vi "Scale Change for Input.vi"(0 "SP:":dbl=34.21052631578948, 1 "Slide Refnum":refnum<vi>, 2 "Slide Refnum 2":refnum<vi>, 3 "WFChart Refnum":refnum<vi>, 5 "Input Unit":enum16{"%", "EGU"}(ring), 7 "Change Scales":bool, 9 "Max In":dbl, 11 "Min In":dbl) -> (4 "SP After Scale Change":dbl=34.21052631578948)   [LabVIEW 2023]
uses:
  <vilib>/addons/control/pid/pid.llb/PID EGU to Percentage (DBL).vi
  <vilib>/addons/control/pid/pid.llb/PID Percentage to EGU (DBL).vi
  <vilib>/addons/control/pid/NI_PID_pid.lvlib
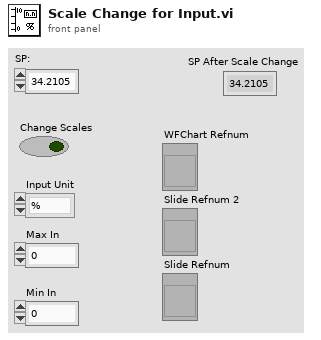
[diagram p1: front panel]
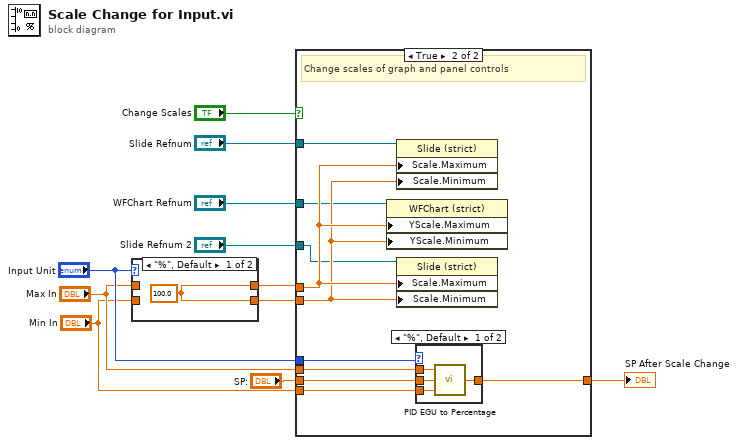
[diagram p0: block diagram]
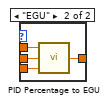
[diagram p3: hidden frame]
diagram:
  n1 = case shown="\"%\", Default" "Input Unit" {
    tunnel: [w12 w14] -> w10
    tunnel: [w12 w13] -> w11
    tunnel: "Max In" -> [_ w14]
    tunnel: "Min In" -> [_ w13]
    frame "%", Default {
      w12 = 100.0 ("Data Range:Maximum")
    }
    frame "EGU" {
    }
  }
  n2 = case shown="True" "Change Scales" {
    tunnel: w10 -> [_ w25]
    tunnel: w11 -> [_ w24]
    tunnel: "Slide Refnum" -> [_ w23]
    tunnel: "Slide Refnum 2" -> [_ w22]
    tunnel: "WFChart Refnum" -> [_ w21]
    tunnel: "SP:" -> [w15 w20]
    tunnel: "Input Unit" -> [_ w19]
    tunnel: [w15 w18] -> w3
    tunnel: "Max In" -> [_ w17]
    tunnel: "Min In" -> [_ w16]
    frame False {
    }
    frame True {
      # "Change scales of graph and panel controls"
      n3 = property on="Property Node" class="WFChart (strict)"(reference=w21, "YScale.Maximum"=w25, "YScale.Minimum"=w24) -> ()  [unwired: 1 in, 2 out]
      n4 = property on="Property Node" class="Slide (strict)"(reference=w23, "Scale.Maximum"=w25, "Scale.Minimum"=w24) -> ()  [unwired: 1 in, 2 out]
      n5 = property on="Property Node" class="Slide (strict)"(reference=w22, "Scale.Maximum"=w25, "Scale.Minimum"=w24) -> ()  [unwired: 1 in, 2 out]
      n6 = case shown="\"%\", Default" w19 {
        tunnel: [w29 w30] -> w18
        tunnel: w20 -> [w28 w32]
        tunnel: w17 -> [w27 w33]
        tunnel: w16 -> [w26 w31]
        frame "%", Default {
          n7 = call-poly <vilib>:"PID EGU to Percentage.vi"("minimum (EGU)"=w26, "input (EGU)"=w28, "maximum (EGU)"=w27) -> ("% span"=w29:dbl)
        }
        frame "EGU" {
          n8 = call-poly <vilib>:"PID Percentage to EGU.vi"("minimum (EGU)"=w31, "% span"=w32, "maximum (EGU)"=w33) -> ("output (EGU)"=w30:dbl)  [unwired: 1 in]
        }
      }
    }
  }
  "SP After Scale Change" <- w3
